vi "Read UserEventReg.vi"(8 "error in (no error)":errorcluster, 11 "SM1000 in":refnum<class "SM1000.lvclass">) -> (0 "error out":errorcluster, 2 "UserEventReg":refnum<event-registration>, 3 "SM1000 out":refnum<class "SM1000.lvclass">)   [LabVIEW 2013, in "SLMControl.lvlib" / "SM1000.lvclass"]
uses:
  SM1000.lvclass
  SM1000.lvclass/SM1000.ctl
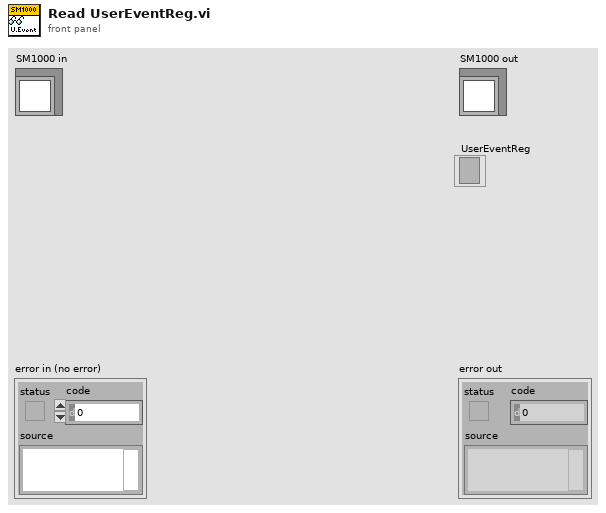
[diagram p1: front panel]
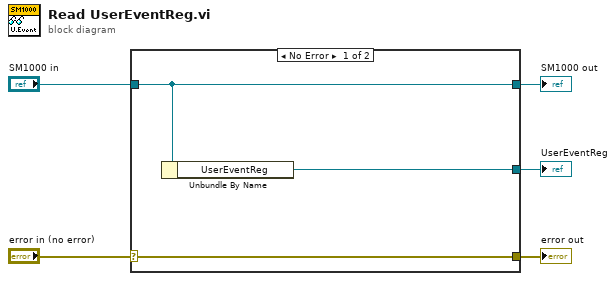
[diagram p0: block diagram]
diagram:
  n1 = case shown="No Error" "error in (no error)" {
    selector: "error in (no error)" -> [w8 w9]
    tunnel: [w8 w9] -> w4
    tunnel: [w7 w10] -> w2
    tunnel: "SM1000 in" -> [w7 w10]
    tunnel: [w6 _] -> w1
    frame No Error {
      n2 = Unbundle By Name(w7) -> ("UserEventReg"=w6:refnum<event-registration>)
    }
    frame Error {
    }
  }
  "error out" <- w4
  "SM1000 out" <- w2
  "UserEventReg" <- w1
